vi "Configure Step Input Trigger Type.vi"(8 "error in (no error)":errorcluster {"code" format="%.0x"}, 9 "TriggerType (I Agxs An 5ss List Sequencer Setup Input Trigger Type Free Run)":i32(ring) items=["I Agxs An 5ss List Sequencer Setup Input Trigger Type Free Run", "I Agxs An 5ss List Sequencer Setup Input Trigger Type Internal", "I Agxs An 5ss List Sequencer Setup Input Trigger Type Manual", "I Agxs An 5ss List Sequencer Setup Input Trigger Type Bus", "I Agxs An 5ss List Sequencer Setup Input Trigger Type External2", "I Agxs An 5ss List Sequencer Setup Input Trigger Type External4"], 10 "StepIndex":i32 format="%.0g", 11 "instrument handle":refnum<k15>) -> (0 "error out":errorcluster {"code" format="%.0x"}, 3 "instrument handle out":refnum<k15>)   [LabVIEW 2009, in "Keysight XSAn.lvlib"]
doc: "Configure the trigger input for the selected step.\n\nSupported Models: M8920A, M9420A, M9421A."
uses:
  <instrlib>/Keysight XSAn/Keysight XSAn.lvlib
  AgXSAn.dll
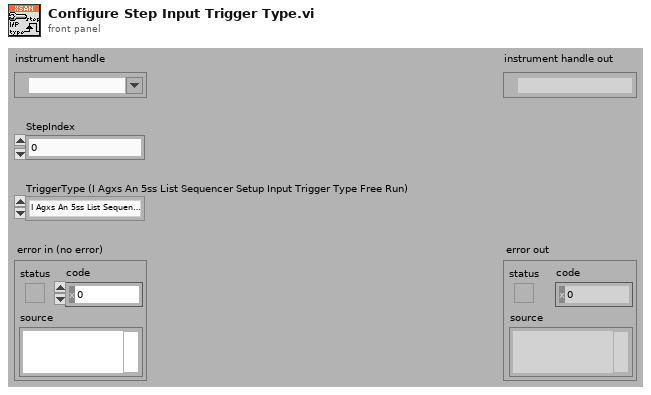
[diagram p1: front panel]
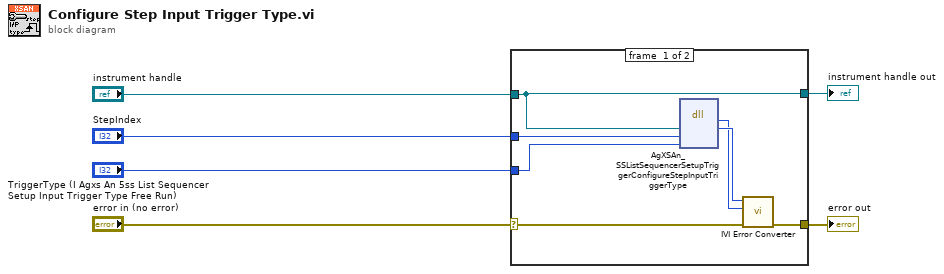
[diagram p0: block diagram]
diagram:
  n1 = case shown="No Error" "error in (no error)" {
    selector: "error in (no error)" -> [w11 w15]
    tunnel: [w10 w15] -> w6
    tunnel: "instrument handle" -> [w7 w14]
    tunnel: "StepIndex" -> [w9 _]
    tunnel: "TriggerType (I Agxs An 5ss List Sequencer Setup Input Trigger Type Free Run)" -> [w8 _]
    tunnel: [w7 w14] -> w1
    frame #0 {
      n2 = dll-call lib="AgXSAn**.dll" fn="AgXSAn_SSListSequencerSetupTriggerConfigureStepInputTriggerType"("Vi"=w7, "StepIndex"=w9, "TriggerType"=w8) -> (w12:i32, "Vi"=w13:u32)  [unwired: 5 in, 2 out]
      n3 = call <instrlib>:"IVI Error Converter.vi"("error in (no error)"=w11, "IVI error code (0)"=w12, "instrument handle"=w13) -> ("error out"=w10:errorcluster)  [unwired: 7 in, 1 out]
    }
    frame #1 {
    }
  }
  "error out" <- w6
  "instrument handle out" <- w1
